vi "DigitalInput Interface.vi"(7 "InputData Refnum":refnum<vi>, 9 "Port index":i32, 11 "Data type":enum16{"State", "Rising", "Falling"}(ring)) -> (2 "Data":bool)   [LabVIEW 2015]
doc: "Interface for accessing the InputData cluster produced by a DigitalInput port type.\n\n\"Port index\": the port address as indexed by the DigitalInput daemon; refer to the port map for detail.\n\"Data type\": what kind of data (State = high/low level of the digital input line as of the last refresh, Rising/Falling = whether a rising/falling edge occurred between refreshes). Default is State."
uses:
  Typedefs/InputData cluster.ctl
  Methods/Port drivers/DigitalInput-DataCluster.ctl
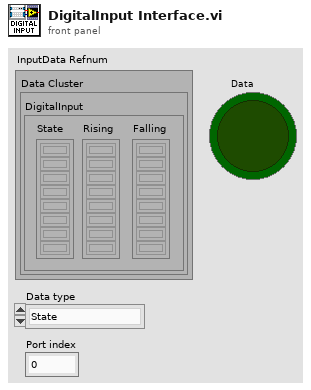
[diagram p1: front panel]
types:
  T1 = typedef "InputData cluster.ctl" = cluster{"DigitalInput":T2}
  T2 = typedef "DigitalInput-DataCluster.ctl" = cluster{"Falling":bool[], "Rising":bool[], "State":bool[]}
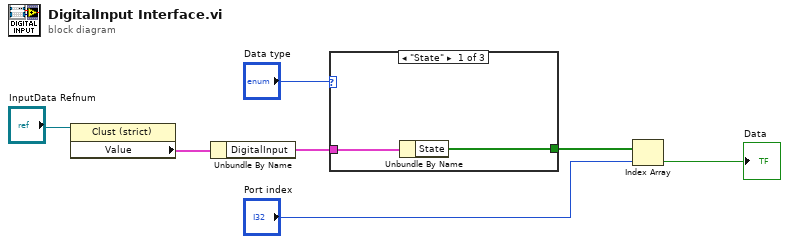
[diagram p0: block diagram]
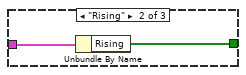
[diagram p2: hidden frame]
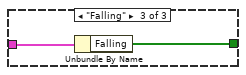
[diagram p3: hidden frame]
diagram:
  n1 = property class="Clust (strict)"(reference="InputData Refnum") -> ("Value"=w2:T1)  [unwired: 1 in, 2 out]
  n2 = Unbundle By Name(w2) -> ("DigitalInput"=w1:T2)
  n3 = case shown="\"State\"" "Data type" {
    tunnel: [w9 w11 w13] -> w6
    tunnel: w1 -> [w8 w10 w12]
    frame "State" {
      n4 = Unbundle By Name(w8) -> ("State"=w9:bool[])
    }
    frame "Rising" {
      n5 = Unbundle By Name(w10) -> ("Rising"=w11:bool[])
    }
    frame "Falling" {
      n6 = Unbundle By Name(w12) -> ("Falling"=w13:bool[])
    }
  }
  n7 = Index Array(array=w6, index="Port index") -> (element=→"Data":bool)
